vi "Map_get.vi"(8 "error in (no error)":errorcluster) -> (0 "error out":errorcluster, 2 "Map":i8[][](array[numeric]))   [LabVIEW 2009, in "NetworkVarTarget.lvlib"]
uses:
  NetworkVarTarget.lvlib
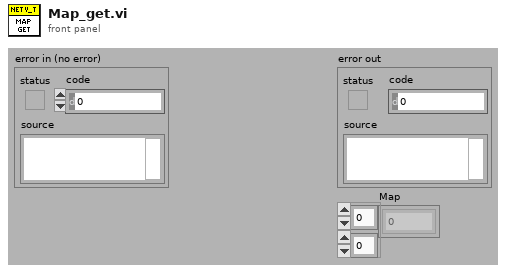
[diagram p1: front panel]
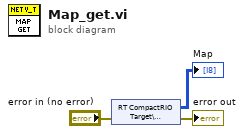
[diagram p0: block diagram]
diagram:
  n1 = shared-variable "RT CompactRIO Target\\NetworkVar.lvlib\\Map"(error in="error in (no error)") -> (→"Map":i8[][], error out=→"error out":errorcluster)
